vi "OAT Polar Update Cursor Name and Position.vi"(6 "precision (2)":i16=2, 9 "X":dbl[](array[numeric]) format="%.2f", 11 "XY Graph":refnum<vi>) -> (2 "cursor positions":dbl[](array[numeric]) format="%.2f")   [LabVIEW 2017]
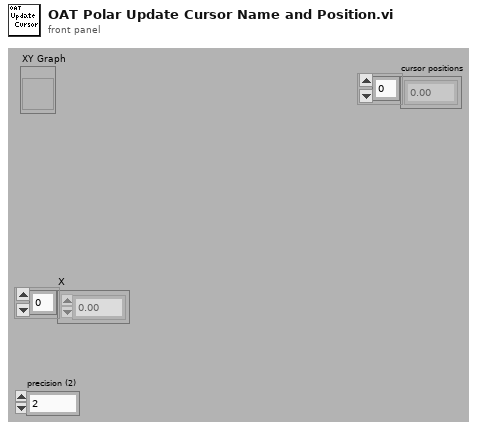
[diagram p1: front panel]
types:
  T1 = cluster{"Name":string, "Color":u32, "Style":u8, "Point Style":u8, "Name Visible":bool, "Allow Drag":bool, "Lock Style":u32, "Plot":u32, "Index":i32, "Position":cluster{"X":dbl, "Y":dbl}}[]
  T2 = cluster{"Name":string, "Color":u32, "Style":u8, "Point Style":u8, "Name Visible":bool, "Allow Drag":bool, "Lock Style":u32, "Plot":u32, "Index":i32, "Position":cluster{"X":dbl, "Y":dbl}}
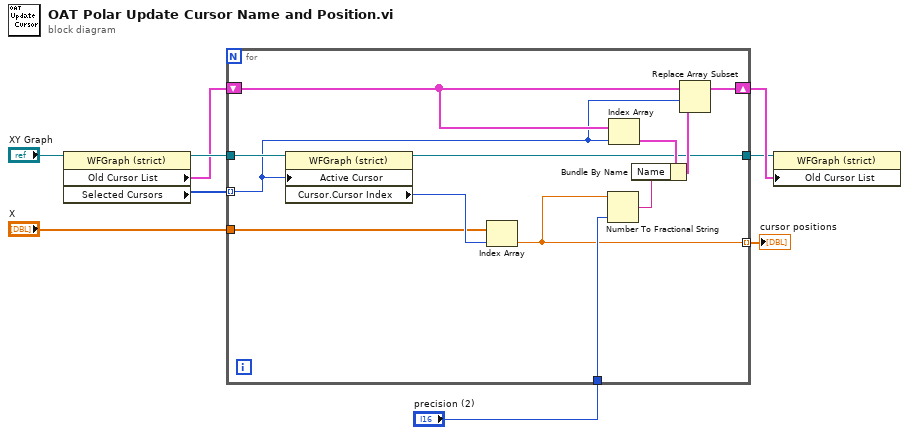
[diagram p0: block diagram]
diagram:
  n1 = property class="WFGraph (strict)"(reference="XY Graph") -> (reference out=w8:refnum<vi>, "Old Cursor List"=w6:T1, "Selected Cursors"=w7:u32[])  [unwired: 1 in, 1 out]
  n2 = for {
    tunnel: w8 -> [w21]
    tunnel: w7 -> [w16] mode=indexing
    shift-right: [w14] -> w4
    shift-left: w6 -> [w17]
    tunnel: "X" -> [w11]
    tunnel: "precision (2)" -> [w20]
    tunnel: [w13] -> w3
    tunnel: [w10] -> w1 mode=indexing
    n3 = property class="WFGraph (strict)"(reference=w21, "Active Cursor"=w16) -> (reference out=w13:refnum<vi>, "Cursor.Cursor Index"=w12:i32)  [unwired: 1 in, 1 out]
    n4 = Index Array(array=w11, index=w12) -> (element=w10:dbl)
    n5 = Number To Fractional String(number=w10, precision (6)=w20) -> (F-format string=w18:string)  [unwired: 2 in]
    n6 = Index Array(array=w17, index=w16) -> (element=w19:T2)
    n7 = Bundle By Name(cluster=w19, "Name"=w18) -> (w15:T2)
    n8 = Replace Array Subset(array=w17, new element=w15, index=w16) -> (w14:T1)
  }
  "cursor positions" <- w1
  n9 = property class="WFGraph (strict)"(reference=w3, "Old Cursor List"=w4) -> ()  [unwired: 1 in, 2 out]
